vi "test16-1ToNBroadcastState.vi"(8 "error in (no error)":errorcluster, 11 "TestCase in":refnum<class "testcase-CSMBroadcast.lvclass">) -> (0 "error out":errorcluster, 3 "TestCase out":refnum<class "testcase-CSMBroadcast.lvclass">)   [LabVIEW 2017, in "testcase-CSMBroadcast.lvclass"]
uses:
  testcase-CSMBroadcast.lvclass
  0b17d103-e67b-41be-a9eb-a2ee1311ff1f.vi
  5999693e-4f8a-4b34-ae87-f34dff5771be.vi
  src/user.lib/_NEVSTOP/Communicable State Machine(CSM)/AdvanceAPI/CSM - Get Module Attribute.vi
  <vilib>/addons/_JKI Toolkits/VI Tester/TestCase.llb/TestCase.lvclass
  src/user.lib/_NEVSTOP/Communicable State Machine(CSM)/Communicable State Machine.lvlib
  CSM/CSM-Testcase.lvlib
  C:/Program Files (x86)/National Instruments/LabVIEW 2017/vi.lib/addons/_JKI Toolkits/VI Tester/TestCase.llb/TestCase.lvclass
panel:
  out "LoopCount2":i32
  out "LoopCount":i32
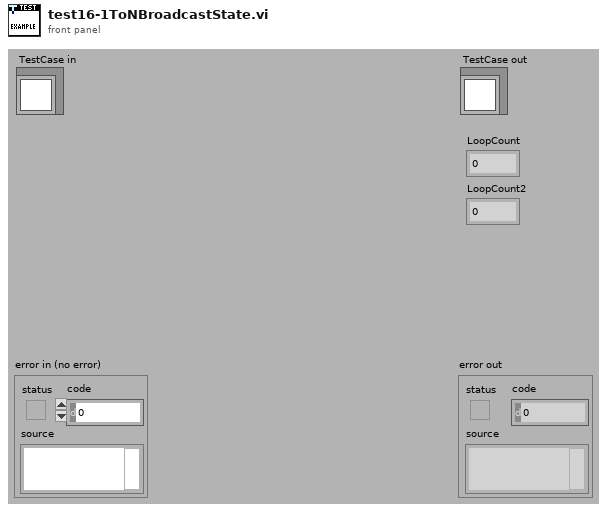
[diagram p1: front panel]
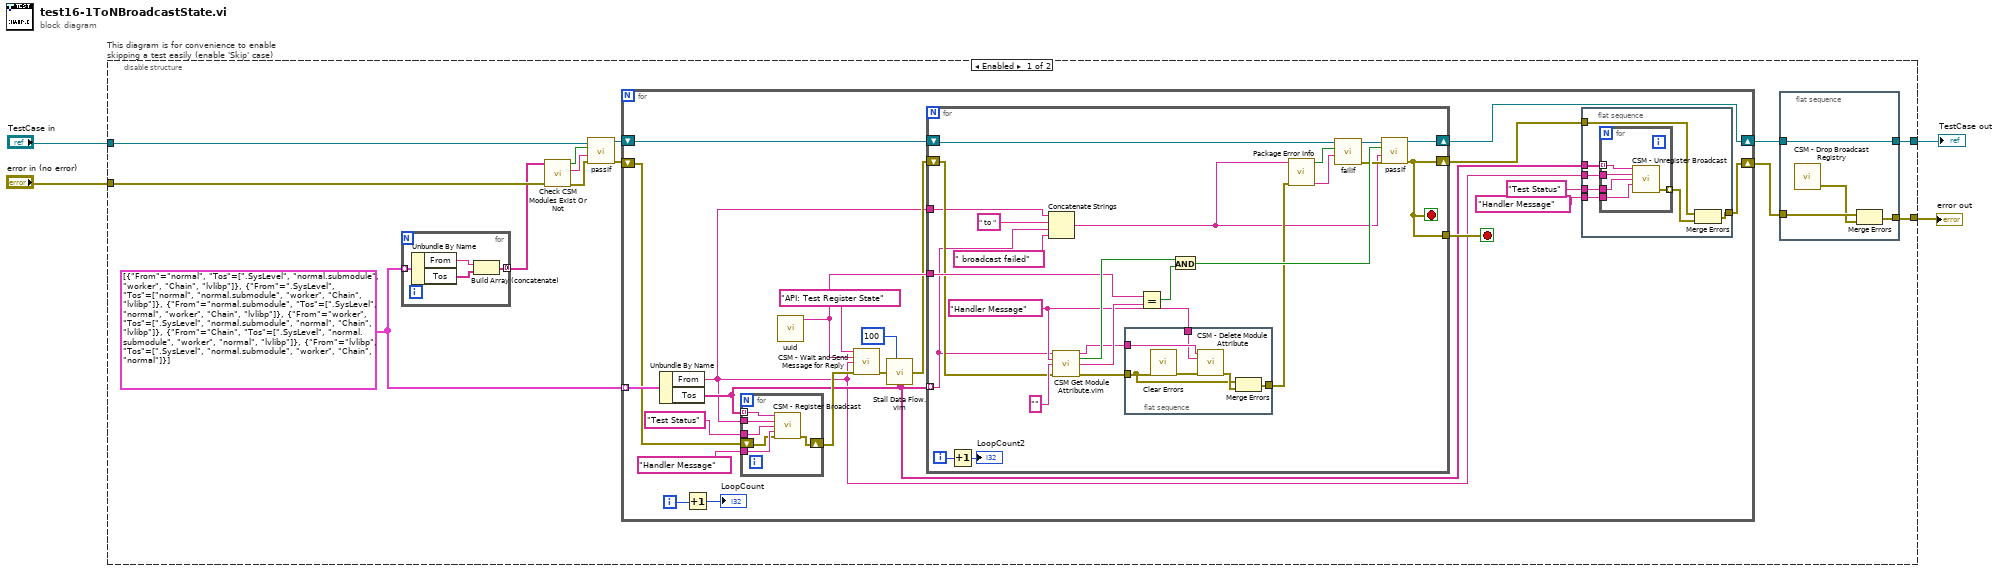
[diagram p0: block diagram]
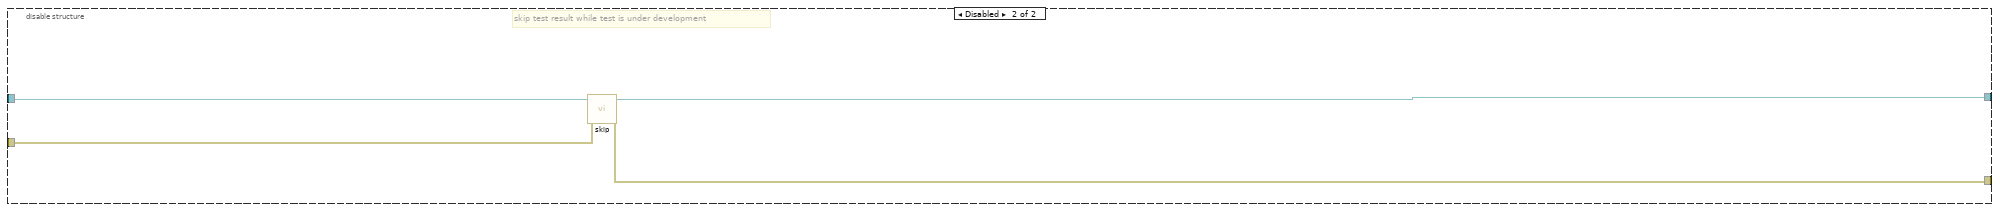
[diagram p2: hidden frame]
diagram:
  n1 = disable-structure "This diagram is for convenience to enable skipping a test easily (enable 'Skip' case)" shown="Enabled" {
    disable-tunnel: "TestCase in" -> [w10 w99]
    disable-tunnel: [w5 w97] -> w1
    disable-tunnel: [w16 w98] -> w3
    disable-tunnel: "error in (no error)" -> [w12 w96]
    frame Enabled {
      w8 = cluster{"From":string, "Tos":string[]}[] [{"From"="normal", "Tos"=[".SysLevel", "normal.submodule", "worker", "Chain", "lvlibp"]}, {"From"=".SysLevel", "Tos"=["normal", "normal.submodule", "worker", "Chain", "lvlibp"]}, {"From"="normal.submodule", "Tos"=[".SysLevel", "normal", "worker", "Chain", "lvlibp"]}, {"From"="worker", "Tos"=[".SysLevel", "normal.submodule", "normal", "Chain", "lvlibp"]}, {"From"="Chain", "Tos"=[".SysLevel", "normal.submodule", "worker", "normal", "lvlibp"]}, {"From"="lvlibp", "Tos"=[".SysLevel", "normal.submodule", "worker", "Chain", "normal"]}]
      n2 = for {
        tunnel: w8 -> [w21] mode=indexing
        tunnel: [w18] -> w7 mode=concatenating
        n3 = Unbundle By Name(w21) -> ("From"=w20:string, "Tos"=w19:string[])
        n4 = Build Array (concatenate)(w20, w19) -> (w18:string[])
      }
      n5 = call "Check CSM Modules Exist Or Not.vi"("error in"=w12, "CSM names in"=w7) -> ("error out"=w13:errorcluster, "Debug string"=w14:string, "All Modules Exist?"=w15:bool)  [unwired: 7 in]
      n6 = call-dynamic "passIf.vi"("error in (no error)"=w13, "message (\"\")"=w14, "pass"=w15, "TestCase in"=w10) -> ("error out"=w11:errorcluster, "TestCase out"=w9:refnum<class "testcase-CSMBroadcast.lvclass">)  [unwired: 6 in]
      n7 = for {
        shift-right: [w34] -> w17
        shift-left: w11 -> [w29]
        shift-right: [w30] -> w6
        shift-left: w9 -> [w39]
        tunnel: w8 -> [w44] mode=indexing
        i -> [w46]
        stop <- w38 stop-if-true
        n8 = Unbundle By Name(w44) -> ("From"=w26:string, "Tos"=w33:string[])
        n9 = Increment(x=w46) -> (x+1=→"LoopCount":i32)
        n10 = for {
          tunnel: w26 -> [w95]
          tunnel: w33 -> [w94] mode=indexing
          tunnel: "Test Status" -> [w93]
          tunnel: "Handler Message" -> [w92]
          shift-right: [w91] -> w35
          shift-left: w29 -> [w90]
          n11 = call "CSM - Register Broadcast.vi"("CSM Name(Empty for Broadcast Event)"=w94, "Source CSM Name (* as Default)"=w95, "Trigger"=w93, "API (If \"\", Same as Trigger)"=w92, "Error In"=w90) -> ("error out"=w91:errorcluster)  [unwired: 9 in, 1 out]
        }
        n12 = call "uuid.vi"() -> ("UUID"=w40:string)  [unwired: 11 in]
        n13 = call "CSM - Wait and Send Message for Reply.vi"("State"="API: Test Register State", "Arguments (\"\")"=w40, "Target Module"=w26, "Error In (No Error)"=w35) -> ("error out"=w42:errorcluster)  [unwired: 8 in, 3 out]
        n14 = call "Stall Data Flow.vim"("value in"=w42, "milliseconds to wait"=u32 100) -> ("value out"=w28:errorcluster)  [unwired: 1 out]
        n15 = for {
          tunnel: w40 -> [w81]
          tunnel: [w70] -> w38
          shift-right: [w79] -> w30
          shift-left: w39 -> [w63]
          shift-right: [w70] -> w27
          shift-left: w28 -> [w71]
          tunnel: w33 -> [w68] mode=indexing
          tunnel: w26 -> [w67]
          i -> [w73]
          stop <- w70 stop-if-true
          w74 = "Handler Message" ("To")
          n16 = Increment(x=w73) -> (x+1=→"LoopCount2":i32)
          n17 = Concatenate Strings(w67, " to " ("string"), w68, " broadcast failed" ("string")) -> (w59:string)
          n18 = call "CSM Get Module Attribute.vim"("CSM Name"=w68, "Attribute"=w74, "Default Value (Empty Variant)"="", "Error In"=w71) -> ("CSM Name (Dup)"=w75:string, "Found"=w83:bool, "Value"=w80:string, "error out"=w76:errorcluster)  [unwired: 7 in, 1 out]
          n19 = flat-sequence {
            tunnel: w76 -> [w85]
            tunnel: w75 -> [w88]
            tunnel: w74 -> [w87]
            tunnel: [w84] -> w60
            frame #0 {
              n20 = call <vilib>:"Clear Errors.vi"("error in (no error)"=w85) -> ("error out"=w89:errorcluster)  [unwired: 5 in, 1 out]
              n21 = call "CSM - Delete Module Attribute.vi"("CSM Name"=w88, "Attribute"=w87, "Error In"=w89) -> ("error out"=w86:errorcluster)  [unwired: 9 in, 3 out]
              n22 = Merge Errors(w85, w86) -> (w84:errorcluster)
            }
          }
          n23 = Equal?(x=w81, y=w80) -> (x = y?=w78:bool)
          n24 = And(x=w83, y=w78) -> (x .and. y?=w77:bool)
          n25 = call "Package Error Info.vi"("error in"=w60, "String in"=w59) -> ("packed error info out"=w64:string, "error status"=w65:bool)  [unwired: 8 in]
          n26 = call-dynamic "failIf.vi"("message (\"\")"=w64, "fail"=w65, "TestCase in"=w63) -> ("error out"=w61:errorcluster, "TestCase out"=w62:refnum<class "testcase-CSMBroadcast.lvclass">)  [unwired: 7 in]
          n27 = call-dynamic "passIf.vi"("error in (no error)"=w61, "message (\"\")"=w59, "pass"=w77, "TestCase in"=w62) -> ("error out"=w70:errorcluster, "TestCase out"=w79:refnum<class "testcase-CSMBroadcast.lvclass">)  [unwired: 6 in]
        }
        n28 = flat-sequence {
          tunnel: [w53] -> w34
          tunnel: w33 -> [w52]
          tunnel: w26 -> [w51]
          tunnel: "Test Status" -> [w50]
          tunnel: "Handler Message" -> [w48]
          tunnel: w27 -> [w47]
          frame #0 {
            n29 = for {
              tunnel: w52 -> [w58] mode=indexing
              tunnel: w51 -> [w57]
              tunnel: w50 -> [w56]
              tunnel: [w55] -> w49 mode=indexing
              tunnel: w48 -> [w54]
              n30 = call "CSM - Unregister Broadcast.vi"("CSM Name(Empty for Broadcast Event)"=w58, "Source CSM Name (* as Default)"=w57, "Trigger"=w56, "API (\"*\" as Default)"=w54) -> ("error out"=w55:errorcluster)  [unwired: 10 in, 1 out]
            }
            n31 = Merge Errors(w47, w49) -> (w53:errorcluster)
          }
        }
      }
      n32 = flat-sequence {
        tunnel: [w25] -> w16
        tunnel: w17 -> [w24]
        tunnel: [w22] -> w5
        tunnel: w6 -> [w22]
        frame #0 {
          n33 = call "CSM - Drop Broadcast Registry.vi"() -> ("error out"=w23:errorcluster)  [unwired: 15 in]
          n34 = Merge Errors(w24, w23) -> (w25:errorcluster)
        }
      }
    }
    frame Disabled {
      # "skip test result while test is under development"
      n35 = call <vilib>:"skip.vi"("error in (no error)"=w96, "TestCase in"=w99) -> ("error out"=w98:errorcluster, "TestCase out"=w97:refnum<class "testcase-CSMBroadcast.lvclass">)  [unwired: 8 in]
    }
  }
  "error out" <- w3
  "TestCase out" <- w1
